vi "Stop-Discard.vi"(4 "queue out":refnum<queue>, 6 "VIRef":refnum<vi>, 7 "Event Common Data":cluster{"Source":T1, "Type":T2, "Time":u32} {"Source" items=["LabVIEW UI"=0, "ActiveX"=1, "User Event"=25]}) -> (0 "Discard?":bool)   [LabVIEW 2021]
uses:
  <vilib>/event_ctls.llb/eventsource.ctl
  <vilib>/event_ctls.llb/lveventtype.ctl
  tdefs/td.Message.ctl
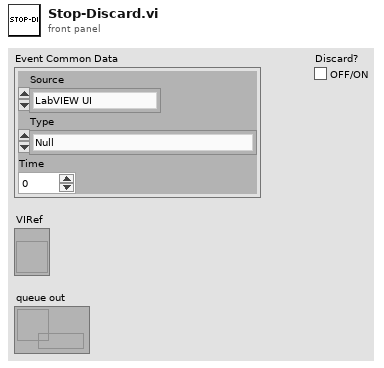
[diagram p1: front panel]
types:
  T1 = typedef "eventsource.ctl" = u32
  T2 = typedef "lveventtype.ctl" = enum32{"Null", "Timeout", "Annotation Menu Selection", "Annotation Menu Selection?", "App Instance Close", "App Instance Close?", "Autoscale Range Change", "Bookmark Info Change", "Cell Edit", "Cell Edit?", "Cursor Grab", "Cursor Grab?", "Cursor Menu Selection", "Cursor Menu Selection?", "Cursor Move", "Cursor Release", "Data Change", "Direction Change", "Display State Change", "Drag Ended", "Drag Enter", "Drag Leave", "Drag Over", "Drag Source Update", "Drag Starting", "Drag Starting?", "Drop", "Exec State Change", "Key Down", "Key Down?", "Key Repeat", "Key Repeat?", "Key Up", "Listbox Double Click", "Menu Activation?", "Menu Selection (App)", "Menu Selection? (App)", "Menu Selection (User)", "Mouse Down", "Mouse Down?", "Mouse Enter", "Mouse Leave", "Mouse Move", "Mouse Up", "Mouse Wheel", "NI Security User Change (App)", "Pane Size", "Panel Close", "Panel Close?", "Panel Resize", "Plot Attribute Change", "Scale Range Change", "Shortcut Menu Activation?", "Shortcut Menu Selection (App)", "Shortcut Menu Selection? (App)", "Shortcut Menu Selection (User)", "Tree Double Click", "Tree Drag", "Tree Drag?", "Tree Drop", "Tree Drop?", "Tree Item Close", "Tree Item Close?", "Tree Item Open", "Tree Item Open?", "User Event", "Value Change"}
  T3 = typedef "td.Message.ctl" = cluster{"Command":string, "Data":variant}
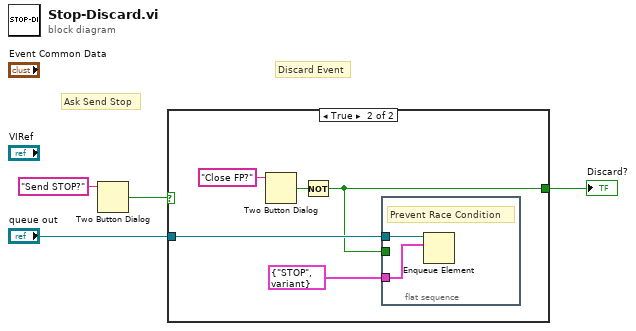
[diagram p0: block diagram]
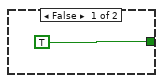
[diagram p2: hidden frame]
diagram:
  # "Discard Event"
  # "Ask Send Stop"
  n1 = Two Button Dialog(message="Send STOP?") -> (T button?=w2:bool)  [unwired: 2 in]
  n2 = case shown="True" w2 {
    tunnel: "queue out" -> [_ w10]
    tunnel: [TRUE w6] -> w1
    frame False {
    }
    frame True {
      n3 = Two Button Dialog(message="Close FP?") -> (T button?=w7:bool)  [unwired: 2 in]
      n4 = Not(x=w7) -> (.not. x?=w6:bool)
      n5 = flat-sequence {
        tunnel: w10 -> [w12]
        tunnel: T3 {"Command"="STOP", "Data"=variant} ("element") -> [w11]
        tunnel: w6 -> [_]
        frame #0 {
          # "Prevent Race Condition"
          n6 = Enqueue Element(queue=w12, element=w11) -> ()  [unwired: 2 in, 3 out]
        }
      }
    }
  }
  "Discard?" <- w1
